vi "hWnd.vi"(10 "VI Refnum":refnum<vi>) -> (2 "hWnd":i32)   [LabVIEW 2020, in "PicoG-Processor.lvlib" / "GVIWebProcessorApp.lvclass"]
uses:
  GVIWebProcessorApp.lvclass
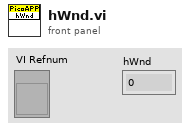
[diagram p1: front panel]
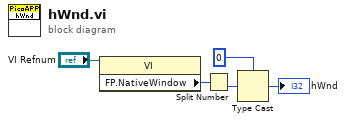
[diagram p0: block diagram]
diagram:
  n1 = property class="VI"(reference="VI Refnum") -> ("FP.NativeWindow"=w5:u64)  [unwired: 1 in, 2 out]
  n2 = Split Number(x=w5) -> (lo(x)=w3:u32)  [unwired: 1 out]
  n3 = Type Cast(type=0, x=w3) -> (*(type *) &x=→"hWnd":i32)
